vi "Edit_Server_Channel.vi"(5 "Mode":T1(ring)) -> ()   [LabVIEW 2014]
uses:
  Sub VIs/ADAM Controls/Ch_description_ADAM.ctl
  Sub VIs/ADAM Controls/Module_type_ADAM.ctl
  Sub VIs/ADAM Controls/Function_ADAM.ctl
  Sub VIs/ADAM Controls/Channel_State.ctl
  Sub VIs/ADAM Controls/Calib_type_ADAM.ctl
  Sub VIs/ADAM Controls/Address.ctl
  Sub VIs/ADAM Controls/Channel_names.ctl
panel:
  out "Help info":string
  in  "Search String":string
  out "Messages":string
  in  "Channel Names":i32(listbox)
  out "String Value":string
  in  "Numerical Value":dbl format="%.11f"
  in  "Ch Description":T2={"Ch Name"="", "Type"="", "Function"=enum."Analogue Input", "Ch State"=enum."On", "Calibration type"=enum."Raw", "A"=0.0, "B"=0.0, "C"=0.0, "D"=0.0, "Comments"="", "Address"={"Main"=0, "Ch."=0, "Sub"=0, "Port Name"=""}, "String"="", "Duty"=65535} {"Duty" format="%.0b"; "D" format="%#_5g"; "C" format="%#_5g"; "B" format="%#_5g"; "A" format="%#_5g"}
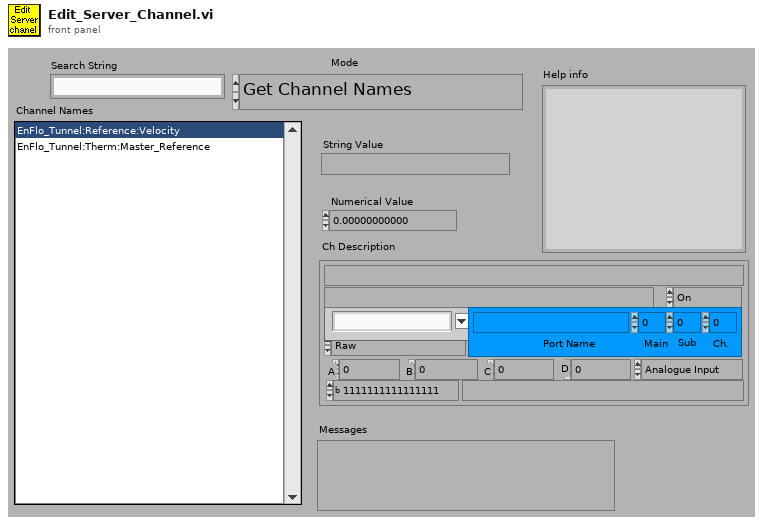
[diagram p1: front panel]
types:
  T1 = enum16{"Get Channel Names", "Get Current Value", "Update Channel Value", "Update Channel Description"}
  T2 = typedef "Ch_description_ADAM.ctl" = cluster{"Ch Name":string, "Type":T3, "Function":T4, "Ch State":T5, "Calibration type":T6, "A":dbl, "B":dbl, "C":dbl, "D":dbl, "Comments":string, "Address":T7, "String":string, "Duty":u16}
  T3 = typedef "Module_type_ADAM.ctl" = string
  T4 = typedef "Function_ADAM.ctl" = enum16{"Analogue Input", "Digital Input", "Event counter", "Event rate", "Analogue Output", "Digital Output", "Relay Output"}
  T5 = typedef "Channel_State.ctl" = enum16{"On", "Off", "Always On", "Always Off"}
  T6 = typedef "Calib_type_ADAM.ctl" = enum16{"Raw", "Bx + A", "Cx^2 + Bx + A", "Dx^3 + Cx^2 + Bx + A", "In Band", "Hi-Tec Q", "Hi-Tec M_dot", "Text"}
  T7 = typedef "Address.ctl" = cluster{"Main":i32, "Ch.":i32, "Sub":i32, "Port Name":string}
  T8 = typedef "Channel_names.ctl" = enum16{"Active Only", "Active + Off", "All Channels"}
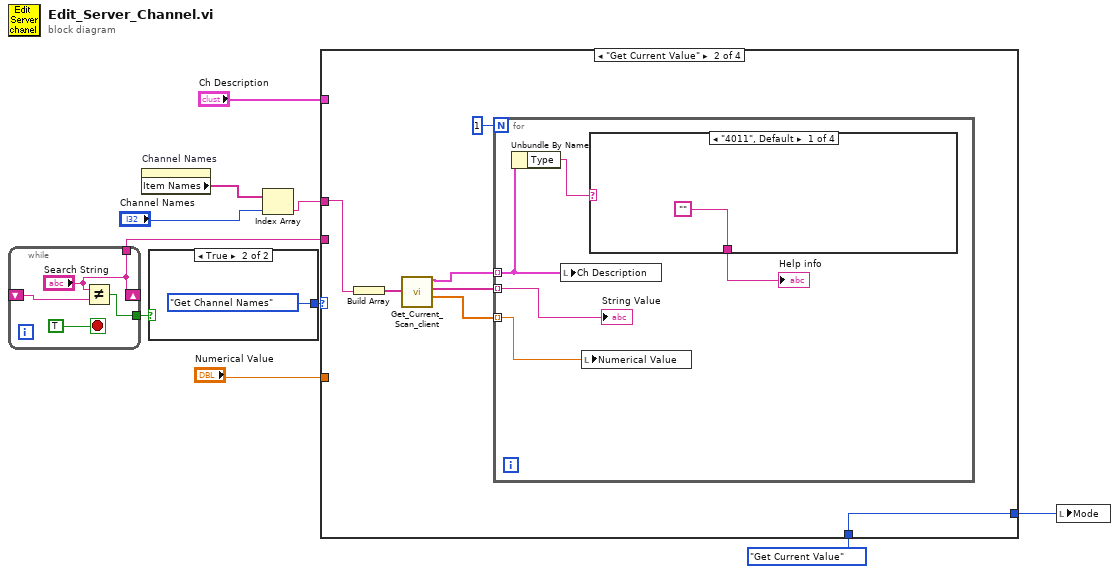
[diagram p0: block diagram]
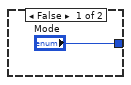
[diagram p2: hidden frame]
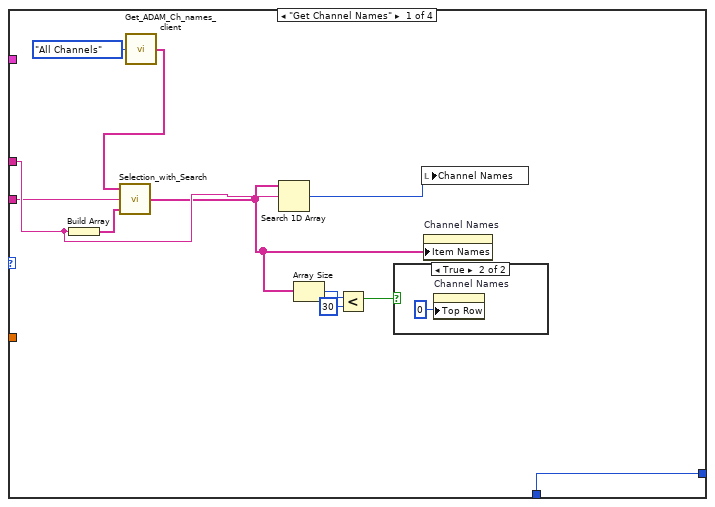
[diagram p3: hidden frame]
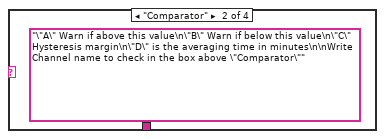
[diagram p5: hidden frame]
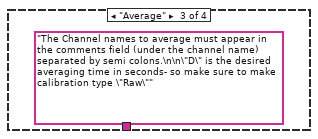
[diagram p6: hidden frame]
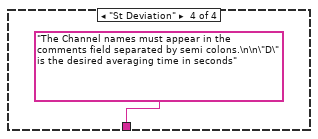
[diagram p7: hidden frame]
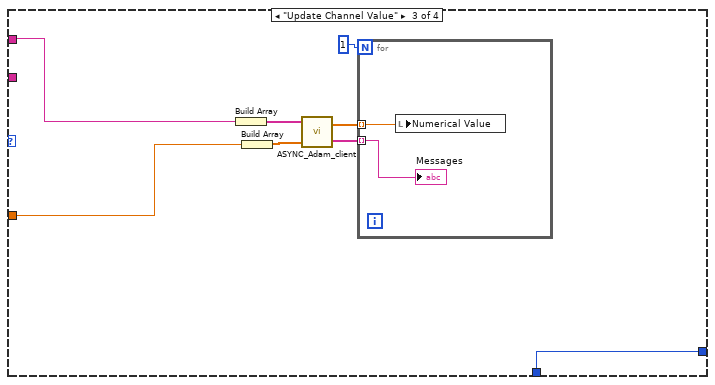
[diagram p8: hidden frame]
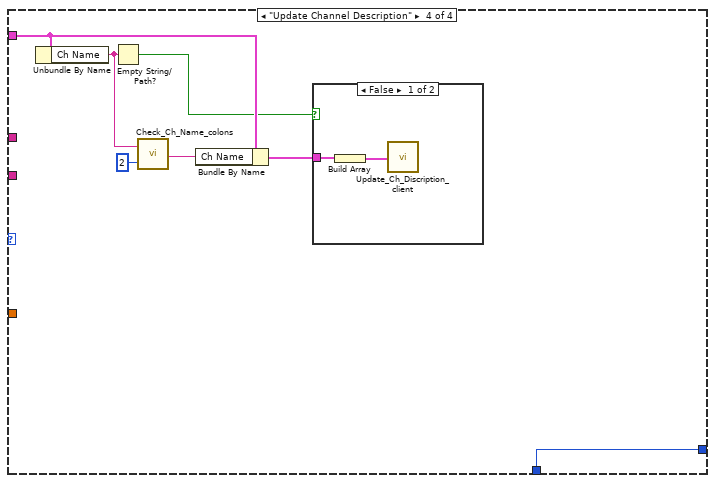
[diagram p9: hidden frame]
diagram:
  n1 = while {
    shift-right: ["Search String"] -> _
    shift-left: _ -> [w14]
    tunnel: [w13] -> w2
    tunnel: ["Search String"] -> w1
    stop <- TRUE stop-if-true
    n2 = Not Equal?(x="Search String", y=w14) -> (x != y?=w13:bool)
  }
  n3 = property on="Channel Names" class="LstBox (strict)"() -> ("Item Names"=w8:string[])  [unwired: 2 in, 2 out]
  n4 = case shown="True" w2 {
    tunnel: ["Mode" T1."Get Channel Names" ("Mode")] -> w10
    frame False {
    }
    frame True {
    }
  }
  n5 = Index Array(array=w8, index="Channel Names") -> (element=w7:string)
  n6 = case shown="\"Get Current Value\"" w10 {
    tunnel: w7 -> [w23 w34 w52 _]
    tunnel: "Numerical Value" -> [_ _ w49 _]
    tunnel: "Ch Description" -> [_ _ _ w60]
    tunnel: T1."Get Current Value" ("Mode") -> [w26 w29 w45 w61]
    tunnel: [w26 w29 w45 w61] -> w3
    tunnel: w1 -> [w21 _ _ _]
    frame "Get Channel Names" {
      n7 = Build Array(w23) -> (w24:string[])
      n8 = call "Get_ADAM_Ch_names_client.vi"("Channel names set"=Channel_names."All Channels") -> ("Ch names"=w25:string[])
      n9 = call "Selection_with_Search.vi"("Selected Channel Names"=w24, "Search String"=w21, "All Channel Names"=w25) -> ("Item Names"=w20:string[])
      n10 = Search 1D Array(1D array=w20, element=w23) -> (index of element=w22:i32)  [unwired: 1 out]
      n11 = Array Size(array=w20) -> (size(s)=w19:i32)
      n12 = Less?(x=w19, y=30) -> (x < y?=w17:bool)
      n13 = case shown="True" w17 {
        frame False {
        }
        frame True {
          n14 = property on="Channel Names" class="LstBox (strict)"("Top Row"=0) -> ()  [unwired: 2 in, 2 out]
        }
      }
      n15 = local write "Channel Names"(w22) -> ()
      n16 = property on="Channel Names" class="LstBox (strict)"("Item Names"=w20) -> ()  [unwired: 2 in, 2 out]
    }
    frame "Get Current Value" {
      n17 = Build Array(w34) -> (w35:string[])
      n18 = call "Get_Current_Scan_client.vi"("ADAM Ch Names"=w35) -> ("Ch Description Array"=w32:T2[], "String values"=w31:string[], "Numerical Values"=w30:dbl[])  [unwired: 1 out]
      n19 = for {
        N: 1 -> [_]
        tunnel: w32 -> [w38] mode=indexing
        tunnel: w31 -> [w40] mode=indexing
        tunnel: w30 -> [w39] mode=indexing
        n20 = Unbundle By Name(w38) -> ("Type"=w37:T3)
        n21 = local write "Ch Description"(w38) -> ()
        n22 = local write "Numerical Value"(w39) -> ()
        n23 = case shown="\"4011\", Default" w37 {
          tunnel: ["" "\"A\" Warn if above this value\n\"B\" Warn if below this value\n\"C\" Hysteresis margin\n\"D\" is the averaging time in minutes\n\nWrite Channel name to check in the box above \"Comparator\"" "The Channel names to average must appear in the comments field (under the channel name) separated by semi colons.\n\n\"D\" is the desired averaging time in seconds- so make sure to make calibration type \"Raw\"" "The Channel names must appear in the comments field separated by semi colons.\n\n\"D\" is the desired averaging time in seconds"] -> w36
          frame "4011", Default {
          }
          frame "Comparator" {
          }
          frame "Average" {
          }
          frame "St Deviation" {
          }
        }
        "Help info" <- w36
        "String Value" <- w40
      }
    }
    frame "Update Channel Value" {
      n24 = Build Array(w52) -> (w51:string[])
      n25 = Build Array(w49) -> (w50:dbl[])
      n26 = call "ASYNC_Adam_client.vi"("Values"=w50, "Channel Names"=w51) -> ("Scan Comments"=w46:string[], "Calibrated Units"=w47:dbl[])  [unwired: 1 in]
      n27 = for {
        N: 1 -> [_]
        tunnel: w47 -> [w54] mode=indexing
        tunnel: w46 -> [w53] mode=indexing
        n28 = local write "Numerical Value"(w54) -> ()
        "Messages" <- w53
      }
    }
    frame "Update Channel Description" {
      n29 = Unbundle By Name(w60) -> ("Ch Name"=w59:string)
      n30 = Empty String/Path?(string/path=w59) -> (empty?=w55:bool)
      n31 = call "Check_Ch_Name_colons.vi"("No of Colons"=2, "Ch Name in"=w59) -> ("Ch Name out"=w57:string)
      n32 = Bundle By Name(cluster=w60, "Ch Name"=w57) -> (w56:T2)
      n33 = case shown="False" w55 {
        tunnel: w56 -> [w62 _]
        frame False {
          n34 = Build Array(w62) -> (w63:T2[])
          n35 = call "Update_Ch_Discription_client.vi"("Channels to update In"=w63) -> ()  [unwired: 1 out]
        }
        frame True {
        }
      }
    }
  }
  n36 = local write "Mode"(w3) -> ()
